vi "EminemGetNoteState.vi"() -> (0 "Box Note State":T1)   [LabVIEW 2023]
uses:
  EminemGlobals.vi
  EminemNoteState.ctl
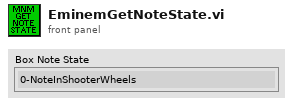
[diagram p1: front panel]
types:
  T1 = typedef "EminemNoteState.ctl" = enum16{"0-NoteInShooterWheels", "1-MisalignedNote", "2-NoNote", "3-HaveNote"}
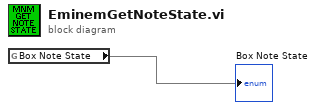
[diagram p0: block diagram]
diagram:
  n1 = global read "EminemGlobals.vi" "Box Note State"() -> (→"Box Note State")
